vi "Cool Down Start.vi"() -> ()   [LabVIEW 2014]
panel:
  out "?":string="Close Me After LabView Starts"
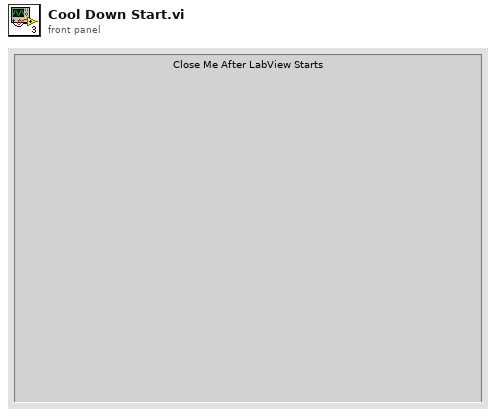
[diagram p1: front panel]
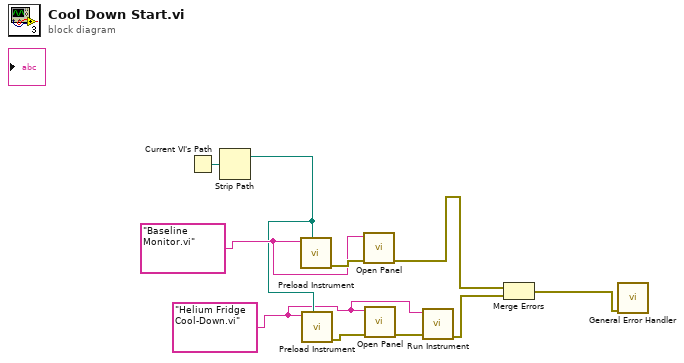
[diagram p0: block diagram]
diagram:
  w4 = "Helium Fridge Cool-Down.vi"
  w8 = "Baseline Monitor.vi"
  n1 = Current VI's Path() -> (path=w10:path)
  n2 = Strip Path(path=w10) -> (stripped path=w5:path)  [unwired: 1 out]
  n3 = call <vilib>:"Preload Instrument.vi"("VI path"=w5, "VI name"=w8) -> ("error out"=w9:errorcluster)  [unwired: 9 in]
  n4 = call <vilib>:"Preload Instrument.vi"("VI path"=w5, "VI name"=w4) -> ("error out"=w7:errorcluster)  [unwired: 9 in]
  n5 = call <vilib>:"Open Panel.vi"("error in (no error)"=w9, "VI name"=w8) -> ("error out"=w1:errorcluster)  [unwired: 9 in]
  n6 = call <vilib>:"Open Panel.vi"("error in (no error)"=w7, "VI name"=w4) -> ("error out"=w6:errorcluster)  [unwired: 9 in]
  n7 = call <vilib>:"Run Instrument.vi"("error in (no error)"=w6, "VI name"=w4) -> ("error out"=w3:errorcluster)  [unwired: 9 in]
  n8 = Merge Errors(w1, w3) -> (w2:errorcluster)
  n9 = call <vilib>:"General Error Handler.vi"("error in (no error)"=w2) -> ()  [unwired: 10 in, 5 out]
